vi "tearDown.vi"(8 "error in (no error)":errorcluster, 11 "reference in":refnum<class "Read Value Tests.lvclass">) -> (0 "error out":errorcluster, 3 "reference out":refnum<class "Read Value Tests.lvclass">)   [LabVIEW 2017, in "Pointer Tests.lvlib" / "Read Value Tests.lvclass"]
doc: "tearDown runs after the test method has completed. Use this method to clean up any operations or references that were opened by setUp or the test method. Unit tests should be independent of other unit tests so this VI should ensure that the next test can run in a 'clean' test environment."
uses:
  Read Value Tests/Read Value Tests.lvclass
  Read Value Tests/Read Value Tests.lvclass/Read Value Tests.ctl
  Source/Classes/Pointer/Pointer.lvclass
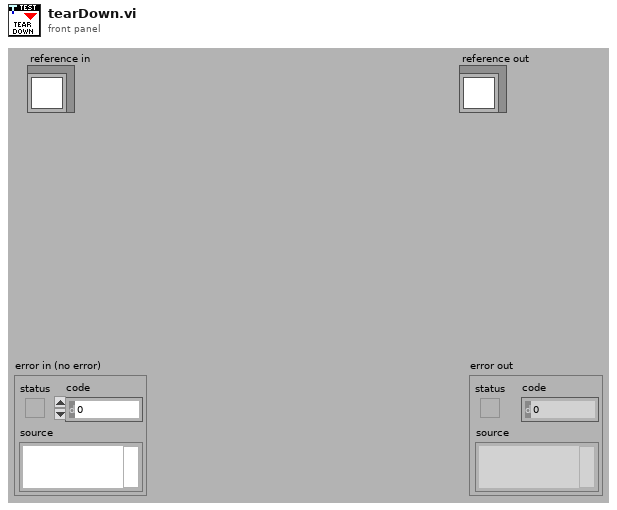
[diagram p1: front panel]
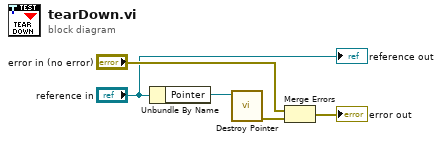
[diagram p0: block diagram]
diagram:
  n1 = Unbundle By Name("reference in") -> ("Pointer"=w2:refnum<class "Pointer.lvclass">)
  n2 = call "Destroy Pointer.vi"("Pointer in"=w2) -> ("error out"=w1:errorcluster)  [unwired: 9 in, 1 out]
  n3 = Merge Errors("error in (no error)", w1) -> (→"error out":errorcluster)
  "reference out" <- "reference in"
